vi "GetDisplayBounds.vi"(8 "error in (no error)":errorcluster) -> (0 "error out":errorcluster, 2 "Dual Monitors":bool, 3 "Display:All Monitors":T1)   [LabVIEW 2015]
uses:
  <vilib>/Utility/miscctls.llb/LVAllMonitorsDisplayTypeDef.ctl
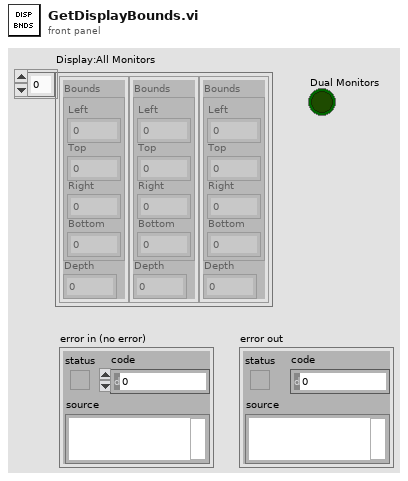
[diagram p1: front panel]
types:
  T1 = typedef "LVAllMonitorsDisplayTypeDef.ctl" = cluster{"Bounds":cluster{"Left":i16, "Top":i16, "Right":i16, "Bottom":i16}, "Depth":i16}[]
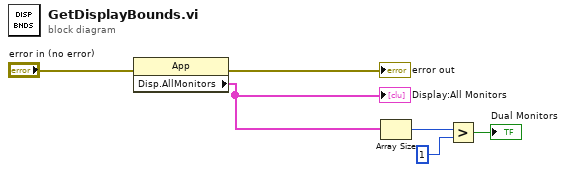
[diagram p0: block diagram]
diagram:
  n1 = property class="App"(error in="error in (no error)") -> (error out=→"error out":errorcluster, "Disp.AllMonitors"=w4:T1)  [unwired: 1 in, 1 out]
  "Display:All Monitors" <- w4
  n2 = Array Size(array=w4) -> (size(s)=w3:i32)
  n3 = Greater?(x=w3, y=1) -> (0:→"Dual Monitors":bool)
